vi "Send Data To FPGA.vi"(6 "Write to FPGA(T)":bool=TRUE, 8 "error in (no error)":errorcluster, 10 "Data":u64[](array[numeric]), 11 "FPGA VI Reference In":refnum<k20>) -> (0 "error out":errorcluster, 3 "FPGA VI Reference Out":refnum<k20>)   [LabVIEW 2016]
uses:
  Typedefs/IO Buffer Operation.ctl
  <vilib>/Utility/error.llb/Error Cluster From Error Code.vi
  <vilib>/rvi/errors/niLvFpgaAdjustHostInterfaceError.vi
  <vilib>/rvi/interface/nirviMethod/nirviMethod.xnode
  <vilib>/FPGAPlugInAG/Dynamic/niLvFpga_WriteFifo_Dynamic.vi
  <vilib>/rvi/errors/niLvFpgaMergeErrorWithErrorCode.vi
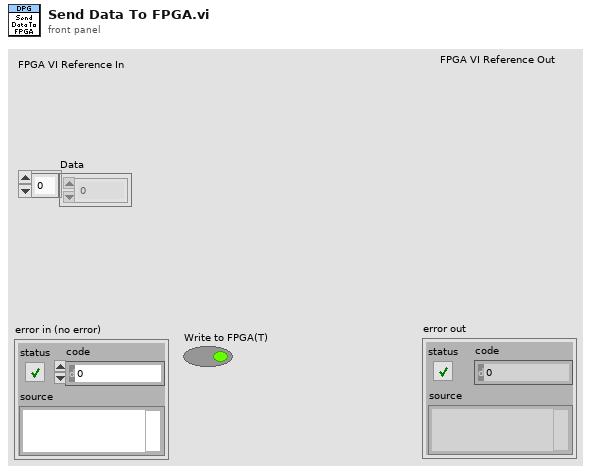
[diagram p1: front panel]
types:
  T1 = typedef "IO Buffer Operation.ctl" = enum16{"Initialize", "Write IO Data_Rd", "Read IO Data_Rd", "Write IO Data_Wr", "Read IO Data_Wr", "Write  IO Data_Dir", "Read  IO Data_Dir", "Write Host to Target FIFO", "Read Host to Target FIFO", "Write Target to Host FIFO", "Read Target to Host FIFO", "Write Monitor Enable?", "Read Monitor Enable?", "Close"}
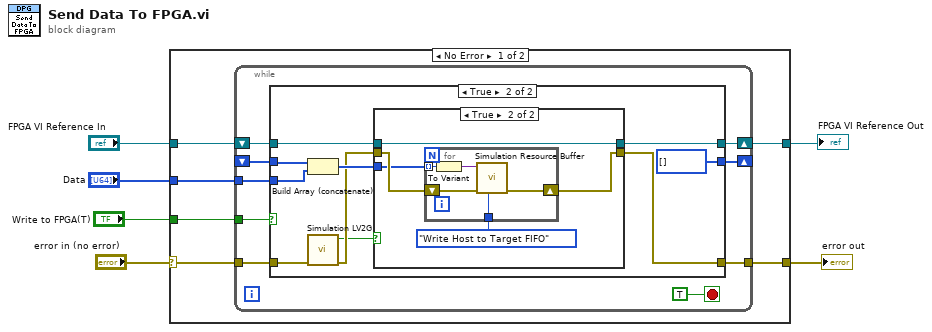
[diagram p0: block diagram]
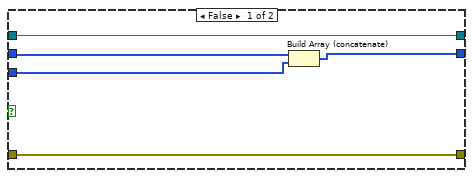
[diagram p2: hidden frame]
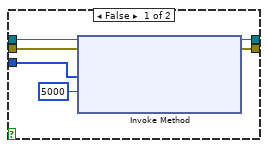
[diagram p3: hidden frame]
diagram:
  n1 = case shown="No Error" "error in (no error)" {
    selector: "error in (no error)" -> [w12 w54]
    tunnel: "FPGA VI Reference In" -> [w11 w53]
    tunnel: [w10 w54] -> w4
    tunnel: "Data" -> [w9 _]
    tunnel: "Write to FPGA(T)" -> [w8 _]
    tunnel: [w7 w53] -> w1
    frame No Error {
      n2 = while {
        tunnel: w12 -> [w21]
        tunnel: [w19] -> w10
        tunnel: w9 -> [w18]
        tunnel: w8 -> [w17]
        shift-right: [w15] -> _
        shift-left: _ -> [w14]
        shift-right: [w13] -> w7
        shift-left: w11 -> [w20]
        stop <- TRUE stop-if-true
        n3 = case shown="True" w17 {
          tunnel: w21 -> [w26 w29]
          tunnel: w20 -> [w22 w36]
          tunnel: [w26 w35] -> w19
          tunnel: w18 -> [w25 w33]
          tunnel: [w24 u64[] []] -> w15
          tunnel: w14 -> [w23 w34]
          tunnel: [w22 w30] -> w13
          frame False {
            n4 = Build Array (concatenate)(w23, w25) -> (w24:u64[])
          }
          frame True {
            n5 = Build Array (concatenate)(w34, w33) -> (w32:u64[])
            n6 = call "Simulation LV2G.vi"("error in (no error)"=w29) -> ("error out"=w28:errorcluster, "Simulation? out"=w27:bool)  [unwired: 9 in]
            n7 = case shown="True" w27 {
              tunnel: w28 -> [w42 w46]
              tunnel: w36 -> [w41 w47]
              tunnel: [w40 w45] -> w35
              tunnel: w32 -> [w38 w43]
              tunnel: [w37 w47] -> w30
              frame False {
                n8 = xnode "Invoke Method"("FPGA VI Reference In"=w41, "error in"=w42, "Data"=w38, "Timeout (ms)"=5000) -> ("FPGA VI Reference Out"=w37:refnum<k20>, "error out"=w40:errorcluster)  [unwired: 1 out]
              }
              frame True {
                n9 = for {
                  tunnel: IO_Buffer_Operation."Write Host to Target FIFO" ("IO Buffer Operation") -> [w50]
                  shift-right: [w51] -> w45
                  shift-left: w46 -> [w52]
                  tunnel: w43 -> [w49] mode=indexing
                  n10 = To Variant(anything=w49) -> (Variant=w48:variant)
                  n11 = call "Simulation Resource Buffer.vi"("IO Buffer Operation"=w50, "error in (no error)"=w52, "Data in"=w48) -> ("error out"=w51:errorcluster)  [unwired: 6 in, 2 out]
                }
              }
            }
          }
        }
      }
    }
    frame Error {
    }
  }
  "error out" <- w4
  "FPGA VI Reference Out" <- w1
